vi "Calcu.vi"() -> ()   [LabVIEW 2019]
panel:
  in  "Stop Button":bool
  out "Display":string
  in  "Botones":T1
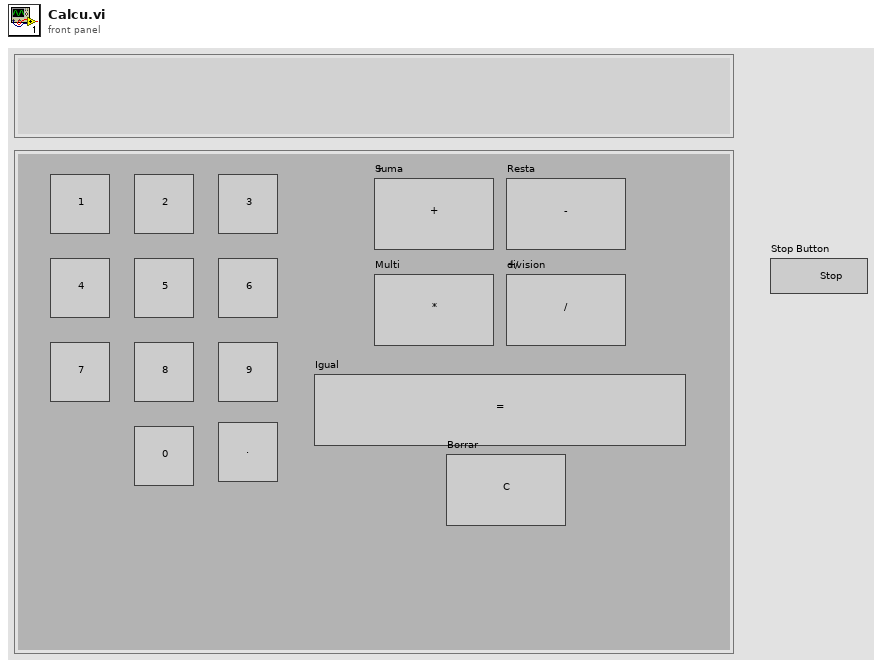
[diagram p1: front panel]
types:
  T1 = cluster{"Uno":bool, "Dos":bool, "Tres":bool, "Cuatro":bool, "Cinco":bool, "Seis":bool, "Siete":bool, "Ocho":bool, "Nueve":bool, "Cero":bool, "Suma":bool, "Resta":bool, "Multi":bool, "division":bool, "Igual":bool, "Borrar":bool, "punti":bool}
  T2 = enum16{"Sin Funcion", "Suma", "Resta", "Multi", "Division"}
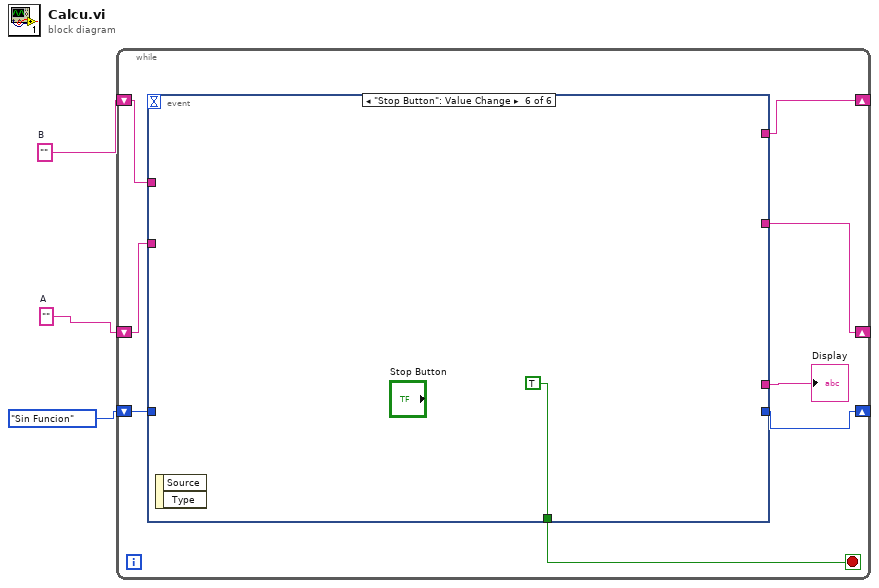
[diagram p0: block diagram]
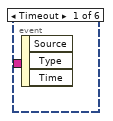
[diagram p2: hidden frame]
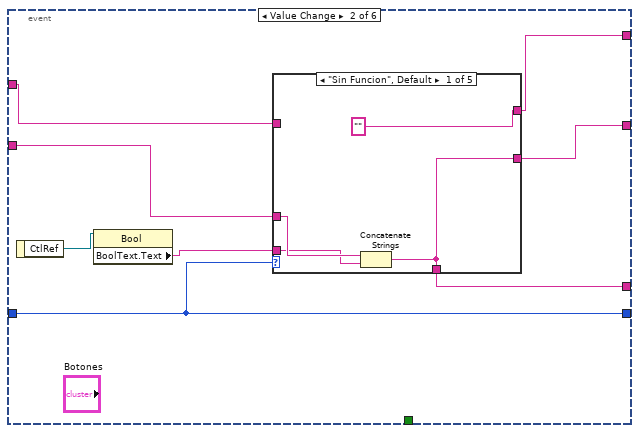
[diagram p3: hidden frame]
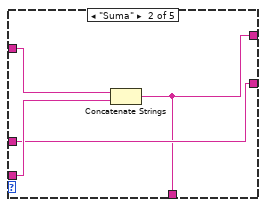
[diagram p4: hidden frame]
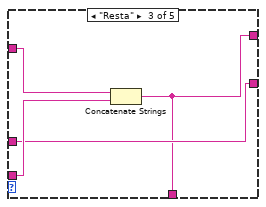
[diagram p5: hidden frame]
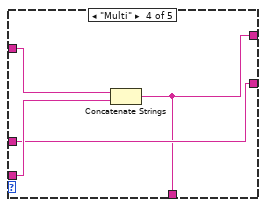
[diagram p6: hidden frame]
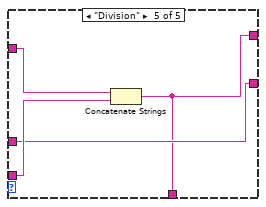
[diagram p7: hidden frame]
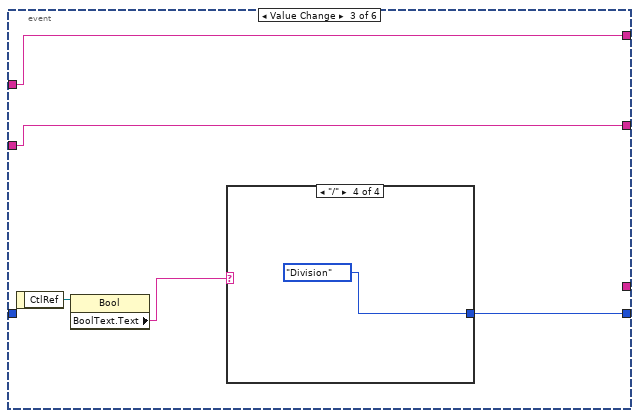
[diagram p8: hidden frame]
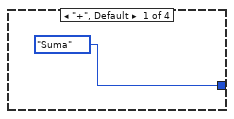
[diagram p9: hidden frame]
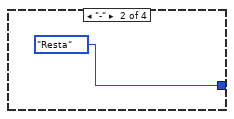
[diagram p10: hidden frame]
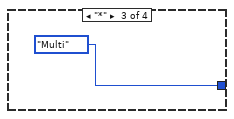
[diagram p11: hidden frame]
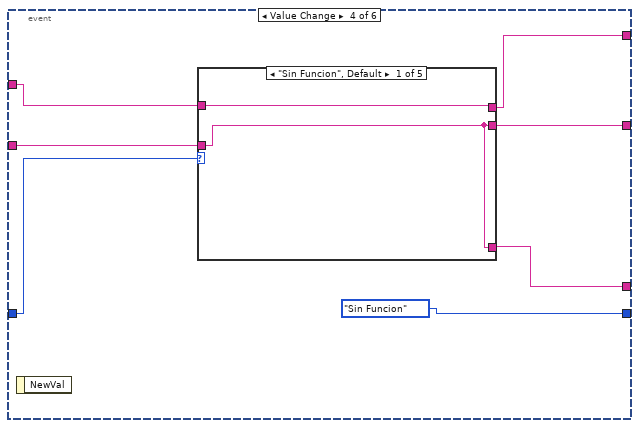
[diagram p12: hidden frame]
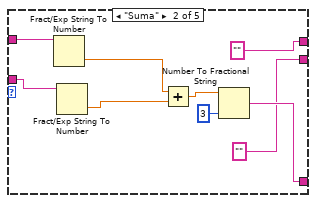
[diagram p13: hidden frame]
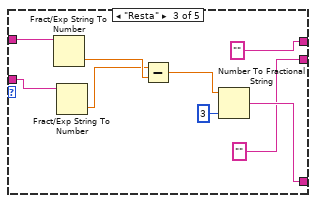
[diagram p14: hidden frame]
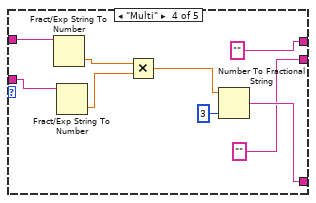
[diagram p15: hidden frame]
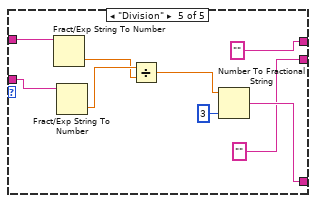
[diagram p16: hidden frame]
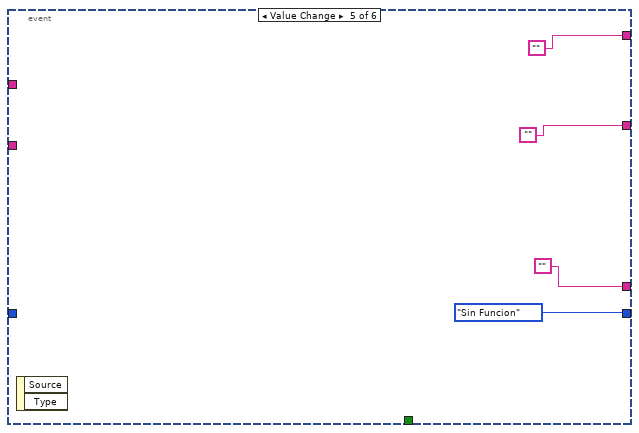
[diagram p17: hidden frame]
diagram:
  w3 = ""  # B
  w2 = ""  # A
  n1 = while {
    shift-right: [w6] -> _
    shift-left: w3 -> [w5]
    shift-right: [w8] -> _
    shift-left: w2 -> [w9]
    shift-right: [w10] -> _
    shift-left: T2."Sin Funcion" -> [w11]
    stop <- w4 stop-if-true
    n2 = event shown="[5] \"Stop Button\": Value Change" {
      selector: _ -> [_ _ _ _ _ _]
      dyn-events: _ -> [_ _ _ _ _ _]
      timeout: _ -> [_ _ _ _ _ _]
      tunnel: w11 -> [_ w19 _ w55 _ _]
      tunnel: [_ w19 w42 T2."Sin Funcion" T2."Sin Funcion" _] -> w10
      tunnel: w9 -> [_ w18 w40 w53 _ _]
      tunnel: [_ w15 w40 w52 "" _] -> w8
      tunnel: [_ w14 _ w49 "" _] -> w7
      tunnel: [_ w13 w41 w50 "" _] -> w6
      tunnel: w5 -> [_ w12 w41 w51 _ _]
      tunnel: [_ _ _ _ _ TRUE] -> w4
      event Timeout {
        n3 = event-data() -> ()  [unwired: 1 in, 3 out]
      }
      event "Botones.punti", "Botones.Uno", "Botones.Dos", "Botones.Tres", "Botones.Cuatro", "Botones.Cinco", "Botones.Seis", "Botones.Siete", "Botones.Ocho", "Botones.Nueve", "Botones.Cero": Value Change {
        n4 = event-data() -> ("CtlRef"=w17:refnum<vi>)  [unwired: 1 in]
        n5 = property class="Bool"(reference=w17) -> ("BoolText.Text"=w16:string)  [unwired: 1 in, 2 out]
        n6 = case shown="\"Sin Funcion\", Default" w19 {
          tunnel: w18 -> [w23 w25 w29 w33 w37]
          tunnel: w16 -> [w22 w26 w30 w34 w38]
          tunnel: [w21 w25 w29 w33 w37] -> w15
          tunnel: [w21 w24 w28 w32 w36] -> w14
          tunnel: ["" w24 w28 w32 w36] -> w13
          tunnel: w12 -> [_ w27 w31 w35 w39]
          frame "Sin Funcion", Default {
            n7 = Concatenate Strings(w23, w22) -> (w21:string)
          }
          frame "Suma" {
            n8 = Concatenate Strings(w27, w26) -> (w24:string)
          }
          frame "Resta" {
            n9 = Concatenate Strings(w31, w30) -> (w28:string)
          }
          frame "Multi" {
            n10 = Concatenate Strings(w35, w34) -> (w32:string)
          }
          frame "Division" {
            n11 = Concatenate Strings(w39, w38) -> (w36:string)
          }
        }
      }
      event "Botones.Suma", "Botones.Resta", "Botones.Multi", "Botones.division": Value Change {
        n12 = event-data() -> ("CtlRef"=w44:refnum<vi>)  [unwired: 1 in]
        n13 = property class="Bool"(reference=w44) -> ("BoolText.Text"=w43:string)  [unwired: 1 in, 2 out]
        n14 = case shown="\"/\"" w43 {
          tunnel: [T2."Suma" T2."Resta" T2."Multi" T2."Division"] -> w42
          frame "+", Default {
          }
          frame "-" {
          }
          frame "*" {
          }
          frame "/" {
          }
        }
      }
      event "Botones.Igual": Value Change {
        n15 = event-data() -> ()  [unwired: 1 in, 1 out]
        n16 = case shown="\"Sin Funcion\", Default" w55 {
          tunnel: w53 -> [w56 w61 w73 w82 w91]
          tunnel: [w56 "" "" "" ""] -> w52
          tunnel: w51 -> [w57 w62 w74 w83 w92]
          tunnel: [w57 "" "" "" ""] -> w50
          tunnel: [w56 w60 w72 w81 w90] -> w49
          frame "Sin Funcion", Default {
          }
          frame "Suma" {
            n17 = Fract/Exp String To Number(string=w62) -> (number=w63:dbl)  [unwired: 3 in, 1 out]
            n18 = Fract/Exp String To Number(string=w61) -> (number=w64:dbl)  [unwired: 3 in, 1 out]
            n19 = Add(x=w63, y=w64) -> (x+y=w65:dbl)
            n20 = Number To Fractional String(number=w65, precision (6)=i16 3) -> (F-format string=w60:string)  [unwired: 2 in]
          }
          frame "Resta" {
            n21 = Fract/Exp String To Number(string=w74) -> (number=w69:dbl)  [unwired: 3 in, 1 out]
            n22 = Fract/Exp String To Number(string=w73) -> (number=w68:dbl)  [unwired: 3 in, 1 out]
            n23 = Subtract(x=w68, y=w69) -> (x-y=w67:dbl)
            n24 = Number To Fractional String(number=w67, precision (6)=i16 3) -> (F-format string=w72:string)  [unwired: 2 in]
          }
          frame "Multi" {
            n25 = Fract/Exp String To Number(string=w83) -> (number=w78:dbl)  [unwired: 3 in, 1 out]
            n26 = Fract/Exp String To Number(string=w82) -> (number=w77:dbl)  [unwired: 3 in, 1 out]
            n27 = Multiply(x=w78, y=w77) -> (x*y=w76:dbl)
            n28 = Number To Fractional String(number=w76, precision (6)=i16 3) -> (F-format string=w81:string)  [unwired: 2 in]
          }
          frame "Division" {
            n29 = Fract/Exp String To Number(string=w92) -> (number=w86:dbl)  [unwired: 3 in, 1 out]
            n30 = Fract/Exp String To Number(string=w91) -> (number=w87:dbl)  [unwired: 3 in, 1 out]
            n31 = Divide(x=w87, y=w86) -> (x/y=w85:dbl)
            n32 = Number To Fractional String(number=w85, precision (6)=i16 3) -> (F-format string=w90:string)  [unwired: 2 in]
          }
        }
      }
      event "Botones.Borrar": Value Change {
        n33 = event-data() -> ()  [unwired: 1 in, 2 out]
      }
      event "Stop Button": Value Change {
        n34 = event-data() -> ()  [unwired: 1 in, 2 out]
      }
    }
    "Display" <- w7
  }
